vi "Password.vi"(8 "error in (no error)":errorcluster, 11 "FTP in":refnum<class "FTP.lvclass">) -> (0 "error out":errorcluster, 3 "FTP out":refnum<class "FTP.lvclass">)   [LabVIEW 2013, in "FTP.lvlib" / "FTP.lvclass"]
uses:
  FTP.lvclass
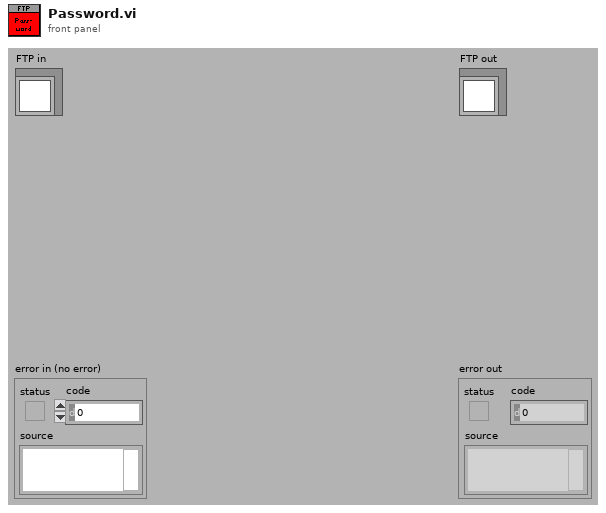
[diagram p1: front panel]
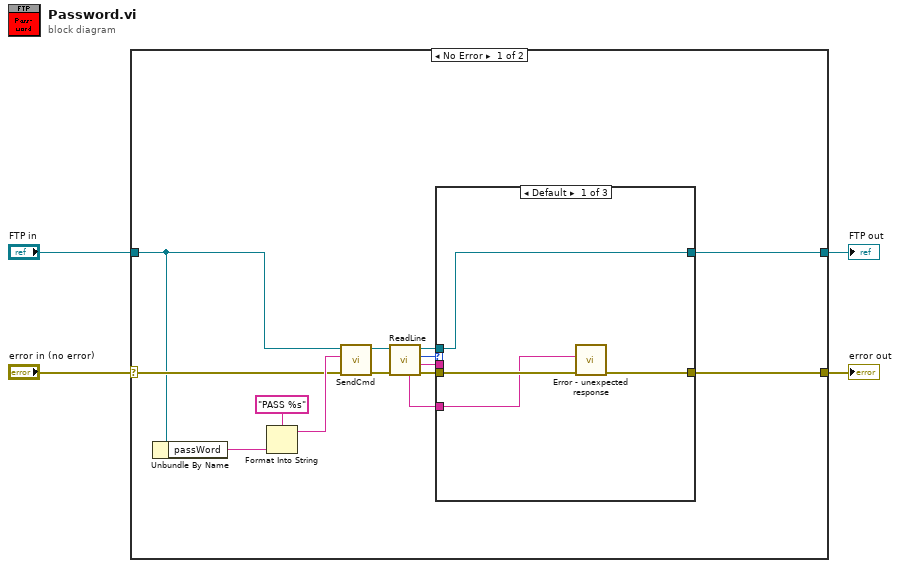
[diagram p0: block diagram]
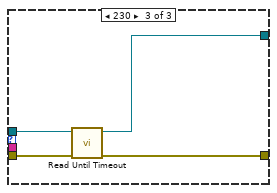
[diagram p3: hidden frame]
diagram:
  n1 = case shown="No Error" "error in (no error)" {
    selector: "error in (no error)" -> [w14 w30]
    tunnel: [w10 w30] -> w3
    tunnel: [w9 w29] -> w1
    tunnel: "FTP in" -> [w7 w29]
    frame No Error {
      n2 = Unbundle By Name(w7) -> ("passWord"=w6:string)
      n3 = Format Into String(format string="PASS %s", w6) -> (resulting string=w16:string)  [unwired: 2 in, 1 out]
      n4 = call "SendCmd.vi"("error in (no error)"=w14, "cmd"=w16, "FTP in"=w7) -> ("error out"=w17:errorcluster, "FTP out"=w18:refnum<class "FTP.lvclass">)  [unwired: 7 in]
      n5 = call "ReadLine.vi"("error in (no error)"=w17, "FTP in"=w18) -> ("error out"=w13:errorcluster, "Line"=w8:string, "code"=w12:i32, "FTP out"=w11:refnum<class "FTP.lvclass">, "Full Line"=w5:string)  [unwired: 5 in]
      n6 = case shown="Default" w12 {
        tunnel: w13 -> [w21 w24 w28]
        tunnel: w11 -> [w22 w23 w27]
        tunnel: [w20 w24 w26] -> w10
        tunnel: [w22 w23 w25] -> w9
        tunnel: w8 -> [_ _ _]
        tunnel: w5 -> [w19 _ _]
        frame Default {
          n7 = call "Error - unexpected response.vi"("error in (no error)"=w21, "Full Response"=w19) -> ("error out"=w20:errorcluster)  [unwired: 9 in]
        }
        frame 202 {
        }
        frame 230 {
          n8 = call "Read Until Timeout.vi"("error in (no error)"=w28, "FTP in"=w27) -> ("error out"=w26:errorcluster, "FTP out"=w25:refnum<class "FTP.lvclass">)  [unwired: 8 in]
        }
      }
    }
    frame Error {
    }
  }
  "error out" <- w3
  "FTP out" <- w1
